vi "FromRepo.vi"(8 "error in":errorcluster, 9 "from repo cluster":T2, 10 "repository in":refnum<class "NISE_CEF_Repository.lvclass">, 11 "Component in":refnum<class "Asynchronous Module Editor Node.lvclass">) -> (0 "error out":errorcluster, 2 "repository out":refnum<class "NISE_CEF_Repository.lvclass">, 3 "node":T1)   [LabVIEW 2013, in "Asynchronous Module Editor Node.lvclass"]
doc: "Grabs information from the Repo and stores it in the nodes."
uses:
  Asynchronous Module Editor Node.lvclass
  <vilib>/CEF_TreeControl/Repository/NISE_CEF_Repository.lvclass
  <vilib>/CEF_TreeControl/Node/FromRepoCluster.ctl
  <vilib>/CEF_TreeControl/Node/NodeRef.ctl
  <vilib>/CEF_TreeControl/Node/NISE_CEF_Node.lvclass
  Configuration Editor/Classes/Module editor node/module editor node.lvclass
  Framework Configuration Classes/platypus configuration/engines cluster.ctl
  <vilib>/NI/Module Execution Interface/Engine Configuration/engine configuration.lvclass
  <vilib>/NI/Tag Bus Module Framework/module configuration/TBM module configuration.lvclass
  configuration/asynchronous execution module configuration.lvclass
  configuration/asynchronous execution module configuration.lvclass/asynchronous execution module configuration.ctl
  Framework Configuration Classes/class cache/class type.ctl
  Configuration Editor/Classes/Module editor node/module editor node.lvclass/module editor node.ctl
  Framework Configuration Classes/class cache/PL_class cache.lvlib
  Framework Configuration Classes/platypus configuration/PLConfigurationSerializer.lvlib
  <vilib>/NI/Tag Bus Module Framework/root configuration/TBM configuration.lvclass
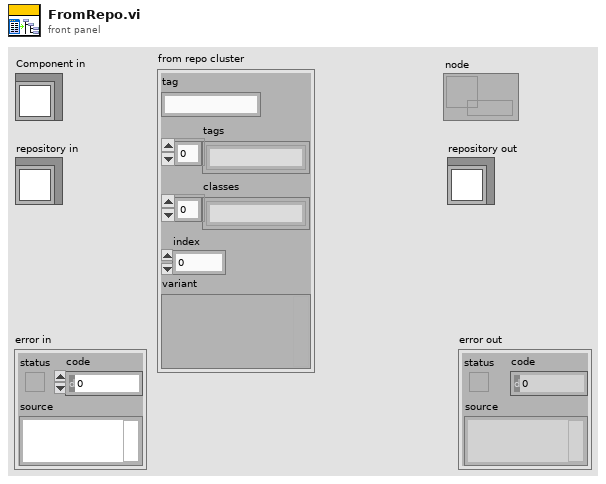
[diagram p1: front panel]
types:
  T1 = typedef "NISE_CEF_Node.lvclass/NodeRef.ctl" = refnum<data-value>
  T2 = typedef "NISE_CEF_Node.lvclass/FromRepoCluster.ctl" = cluster{"tag":string, "tags":string[], "classes":string[], "index":i32, "variant":variant}
  T3 = typedef "PLConfigurationSerializer.lvlib/engines cluster.ctl" = cluster{"engine configuration":refnum<class "engine configuration.lvclass">, "modules":refnum<class "TBM module configuration.lvclass">[]}
  T4 = typedef "PL_class cache.lvlib/class type.ctl" = enum16{"unused", "target", "engine", "module"}
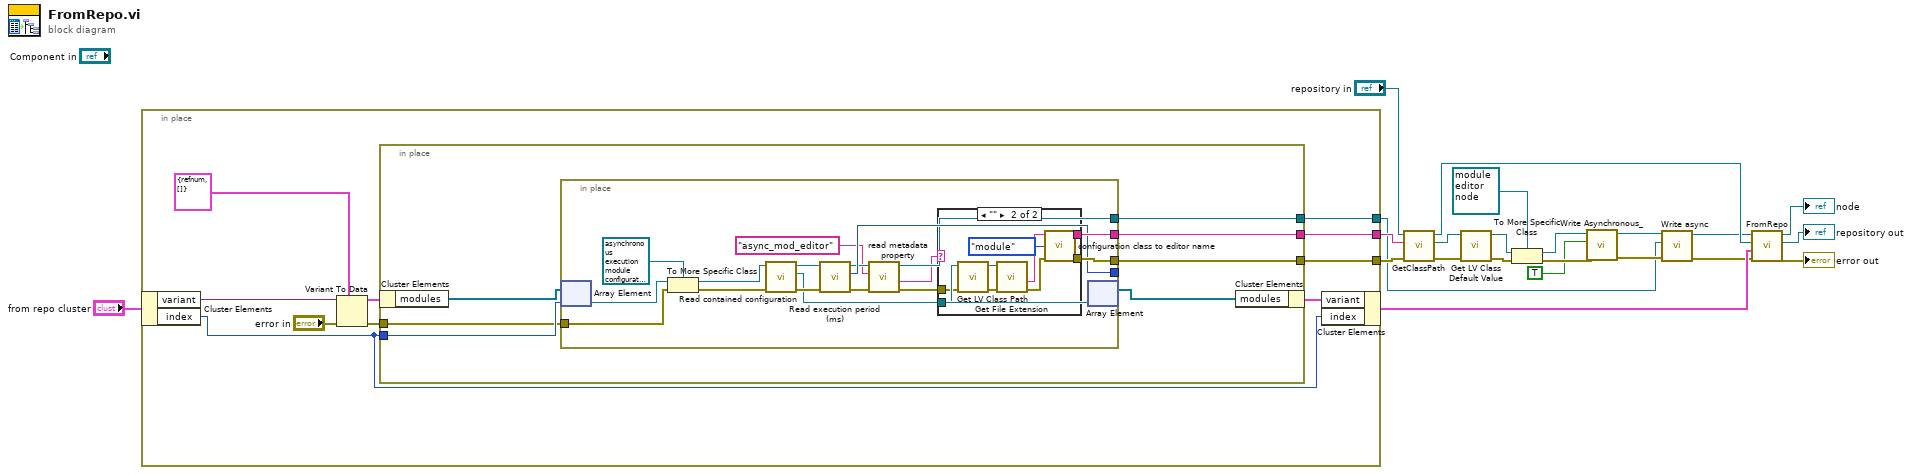
[diagram p0: block diagram]
diagram:
  n1 = in-place {
    in-place-border: [w30] -> w21
    in-place-border: [w29] -> w12
    in-place-border: [w23] -> w1
    n2 = in-place-cluster #1("from repo cluster") -> ("variant"=w27:variant, "index"=w25:i32)
    n3 = Variant To Data(error in="error in", type=T3 {"engine configuration"=refnum, "modules"=[]} ("engines cluster"), Variant=w27) -> (data=w32:T3, error out=w28:errorcluster)
    n4 = in-place {
      in-place-border: w25 -> [w37]
      in-place-border: [w36] -> w30
      in-place-border: [w35] -> w29
      in-place-border: w28 -> [w34]
      in-place-border: [w33] -> w23
      n5 = in-place-cluster #2(w32) -> ("modules"=w39:refnum<class "TBM module configuration.lvclass">[])
      n6 = in-place {
        in-place-border: [w54] -> w36
        in-place-border: [w53] -> w35
        in-place-border: w34 -> [w52]
        in-place-border: [w49] -> _
        in-place-border: [w44] -> w33
        n7 = in-place-array #3(w39, w37) -> (w56:refnum<class "TBM module configuration.lvclass">)
        n8 = To More Specific Class(target class=refnum<class "asynchronous execution module configuration.lvclass"> refnum ("Asynchronous Component Configuration"), reference=w56, error in=w52) -> (specific class reference=w46:refnum<class "asynchronous execution module configuration.lvclass">, error out=w45:errorcluster)
        n9 = call "Read contained configuration.vi"("error in"=w45, "asynchronous execution module configuration in"=w46) -> ("error out"=w51:errorcluster, "module configuration"=w48:refnum<class "TBM module configuration.lvclass">, "asynchronous execution module configuration out"=w50:refnum<class "asynchronous execution module configuration.lvclass">)  [unwired: 7 in]
        n10 = call "Read execution period (ms).vi"("error in"=w51, "Asynchronous Component Configuration in"=w50) -> ("error out"=w43:errorcluster, "execution period (ms)"=w49:i32, "Asynchronous Component Configuration out"=w47:refnum<class "asynchronous execution module configuration.lvclass">)  [unwired: 7 in]
        n11 = call <vilib>:"read metadata property.vi"("error in"=w43, "key"="async_mod_editor", "configuration in"=w47) -> ("error out"=w42:errorcluster, "value"=w40:string, "configuration out"=w44:refnum<class "asynchronous execution module configuration.lvclass">)  [unwired: 5 in, 1 out]
        n12 = case shown="\"\"" w40 {
          selector: w40 -> [w57 _]
          tunnel: [w57 w67] -> w54
          tunnel: [w58 w66] -> w53
          tunnel: w48 -> [_ w63]
          tunnel: w42 -> [w58 w59]
          frame Default {
          }
          frame "" {
            n13 = call <vilib>:"Get LV Class Path.vi"("error in (no error)"=w59, "object"=w63) -> ("error out"=w65:errorcluster, "class path"=w61:path)  [unwired: 8 in]
            n14 = call <vilib>:"Get File Extension.vi"("error in (no error)"=w65, "file"=w61) -> ("error out"=w62:errorcluster, "filename without extension"=w60:string)  [unwired: 6 in, 2 out]
            n15 = call "configuration class to editor name.vi"("class type"=class_type."module", "error in"=w62, "configuration class name"=w60) -> ("error out"=w66:errorcluster, "editor node class name"=w67:string)  [unwired: 7 in]
          }
        }
        n16 = in-place-array #3(w48) -> (w38:refnum<class "TBM module configuration.lvclass">[])  [unwired: 1 out]
      }
      n17 = in-place-cluster #2("modules"=w38) -> (w26:T3)
    }
    n18 = in-place-cluster #1("variant"=w26, "index"=w25) -> (w9:T2)
  }
  n19 = call-dynamic "GetClassPath.vi"("error in"=w12, "class name"=w21, "Repository in"="repository in") -> ("error out"=w22:errorcluster, "class path"=w20:path, "Repository out"=w18:refnum<class "NISE_CEF_Repository.lvclass">)  [unwired: 6 in]
  n20 = call <vilib>:"Get LV Class Default Value.vi"("error in (no error)"=w22, "class path"=w20) -> ("error out"=w14:errorcluster, "object"=w16:refnum<class>)  [unwired: 8 in]
  n21 = To More Specific Class(target class=refnum<class "module editor node.lvclass"> refnum ("Component Parent.lvclass"), reference=w16, error in=w14) -> (specific class reference=w3:refnum<class "module editor node.lvclass">, error out=w7:errorcluster)
  n22 = call-dynamic "Write Asynchronous_.vi"("error in"=w7, "Asynchronous?"=TRUE ("Asynchronous_"), "Module Editor Node in"=w3) -> ("error out"=w6:errorcluster, "Module Editor Node out"=w8:refnum<class "module editor node.lvclass">)  [unwired: 7 in]
  n23 = call "Write async.vi"("error in"=w6, "async module"=w1, "module editor node in"=w8) -> ("error out"=w5:errorcluster, "module editor node out"=w4:refnum<class "module editor node.lvclass">)  [unwired: 7 in]
  n24 = call-dynamic "FromRepo.vi"("error in"=w5, "from repo cluster"=w9, "repository in"=w18, "module editor node in"=w4) -> ("error out"=→"error out":errorcluster, "repository out"=→"repository out":refnum<class "NISE_CEF_Repository.lvclass">, "module editor node out"=→"node":T1)  [unwired: 5 in]
